vi "maze_v3.vi"   [LabVIEW 2012]
uses:
  <vilib>/NXT/Subs/MotorOutput.ctl
  <vilib>/NXT/Block Support/NXT_InputPort.ctl
  <vilib>/NXT/Dual Mode Library/Motors/MotorReverse.vi
  <vilib>/NXT/Dual Mode Library/Motors/MotorOn.vi
  <vilib>/NXT/Dual Mode Library/Motors/MotorBrake.vi
  <vilib>/NXT/Dual Mode Library/Display/clearDisplay.vi
  <vilib>/NXT/Dual Mode Library/Display/drawText.vi
  <vilib>/NXT/Dual Mode Library/Waits/Wait_Num(msec).vi
  <vilib>/NXT/Dual Mode Library/Display/drawLine.vi
  <vilib>/NXT/Dual Mode Library/Waits/Wait_Num.vi
  <vilib>/NXT/Dual Mode Library/Display/drawNumber.vi
types:
  T1 = typedef "MotorOutput.ctl" = u8
  T2 = typedef "LVHSConnector.ctl" = cluster{"Hardware":string, "Flattened String":string}
  T3 = typedef "NXT_InputPort.ctl" = u8
  T4 = cluster{"x-y*floor(x/y)":i32, "Start X":i16, "x-y*floor(x/y)":i32, i16}
  T5 = cluster{"x":i32, "Start X":i16, "x":i32, "Start X":i16}
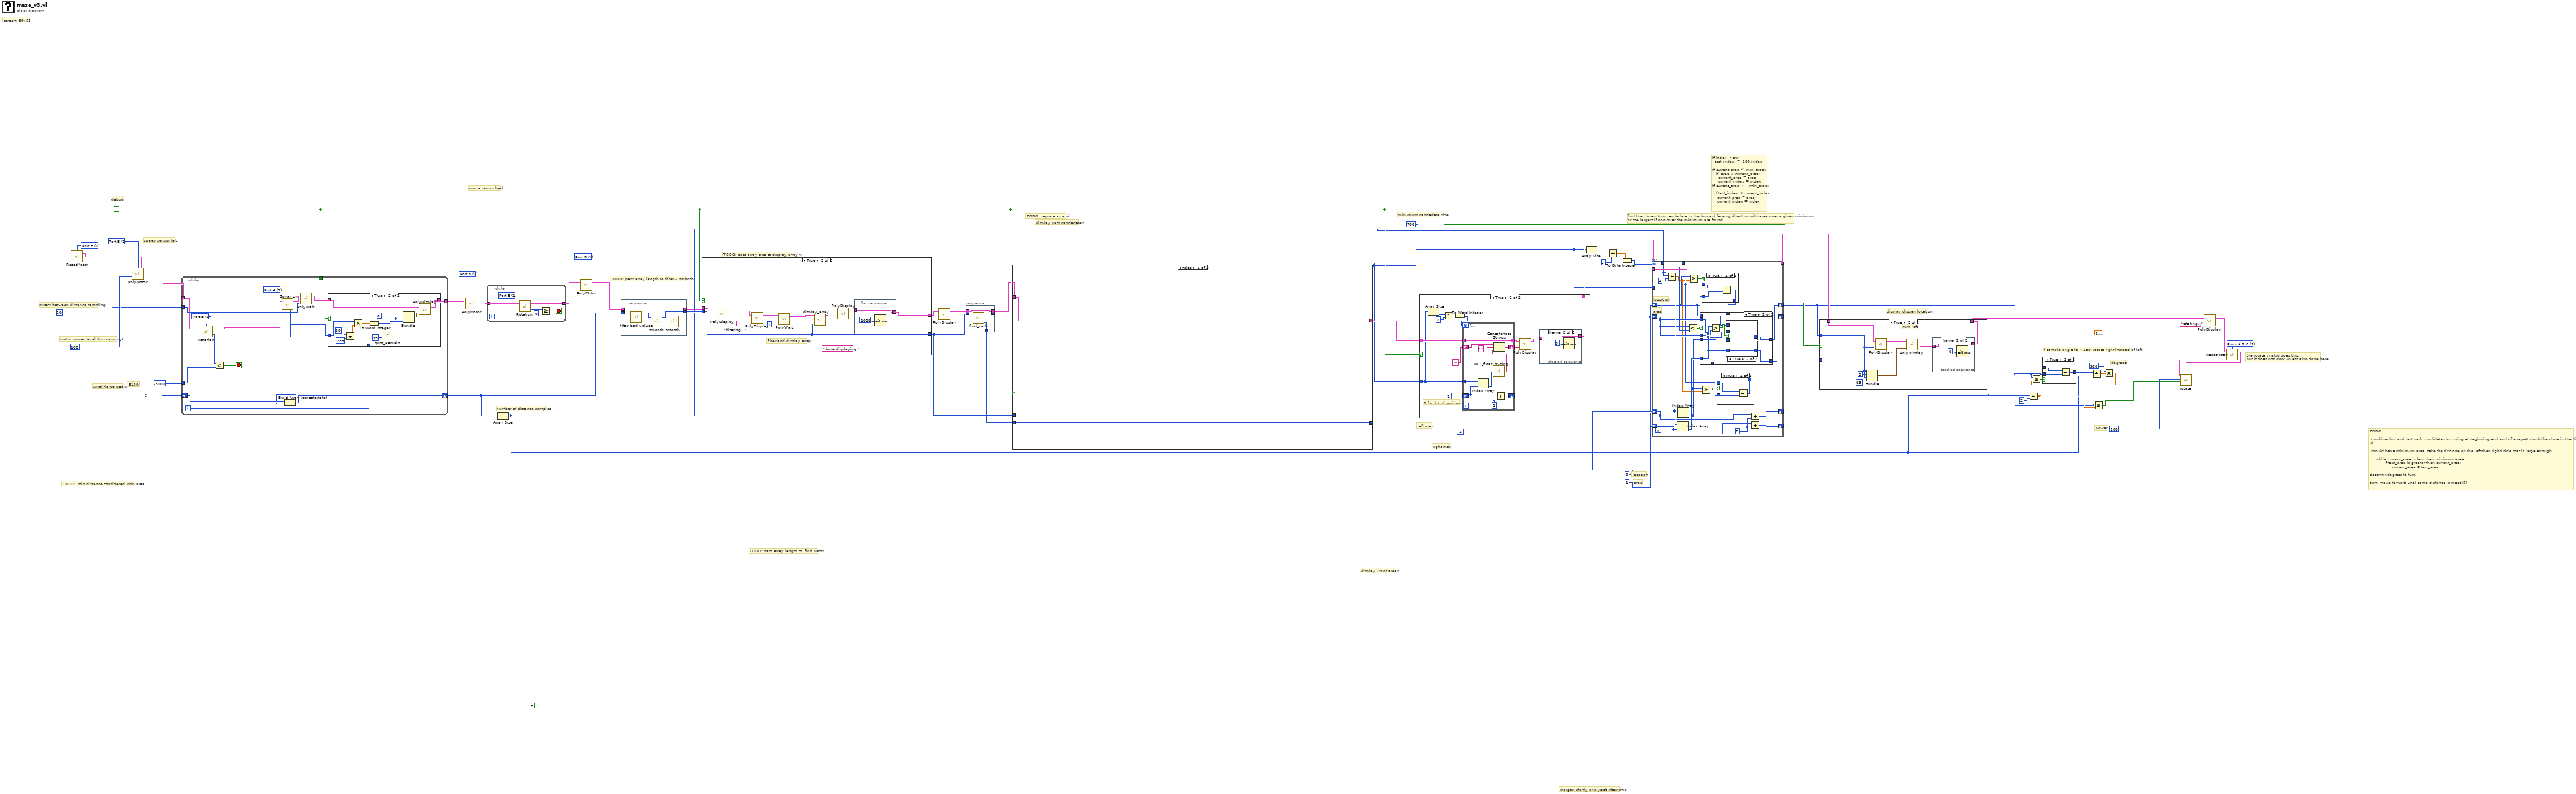
[diagram p0: block diagram]
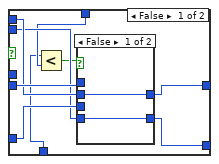
[diagram p9: hidden frame]
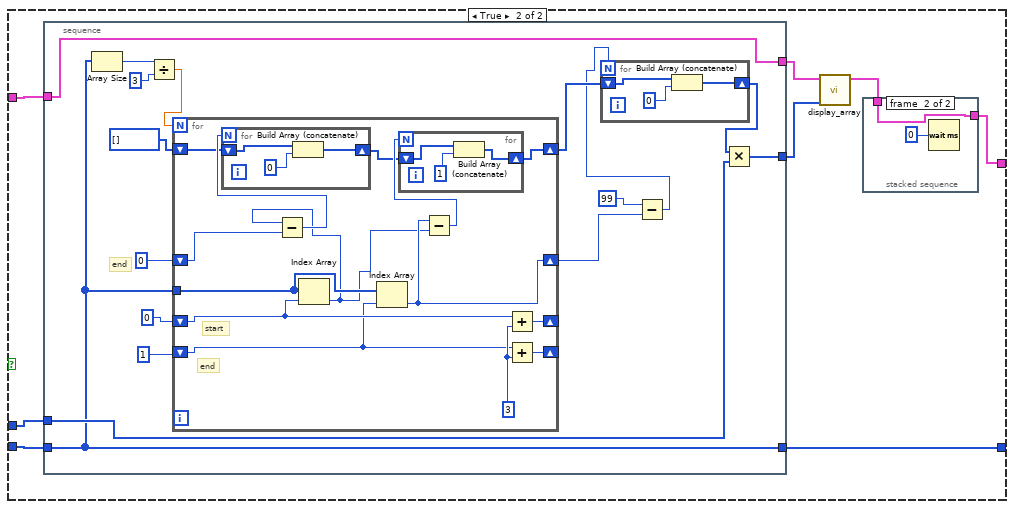
[diagram p13: hidden frame]
diagram:
  w13 = T1 1 items=["Port A"=0, "Port B"=1, "Port C"=2, "Ports A & B"=4, "Ports A & C"=5, "Ports B & C"=6, "as"=3] ("Output Port (All Ports)")
  w14 = T1 1 items=["Port A"=0, "Port B"=1, "Port C"=2, "Ports A & B"=4, "Ports A & C"=5, "Ports B & C"=6, "as"=3] ("Output Port (All Ports)")
  w21 = T1 1 items=["Port A"=0, "Port B"=1, "Port C"=2, "Ports A & B"=4, "Ports A & C"=5, "Ports B & C"=6, "All Ports"=3] ("Port (All Ports)")
  w25 = T1 5 items=["Port A"=0, "Port B"=1, "Port C"=2, "Ports A & B"=4, "Ports A & C"=5, "Ports B & C"=6, "All Ports"=3] ("Port (All Ports)")
  (unwired) 6.283185307179586 ("Pi Multiplied By 2")
  w37 = i16 -1 ("Start X")
  (unwired) FALSE
  w35 = TRUE
  w52 = T1 1 items=["Port A"=0, "Port B"=1, "Port C"=2, "Ports A & B"=4, "Ports A & C"=5, "Ports B & C"=6, "as"=3] ("Output Port (All Ports)")
  # "small-large gears"
  # "-5100"
  # "sweep sensor left"
  # "move sensor back"
  # "if sample angle is > 180, rotate right instead of left"
  # "TODO: pass array length to  find paths"
  # "TODO: pass array size to display array vi"
  # "TODO: pass array length to filter & smooth"
  # "number of distance samples"
  # "the rotate vi also does this,\nbut it does not work unless also done here"
  # "power"
  # "degrees"
  # "display chosen location"
  # "display list of areas"
  # "if index > 50;\n  test_index  =  100-index\n\nif current_area <  min_area:\n   if  area > current_area:\n     current_area = area\n     current_index = index\nif current_area >=  min_area:\n\n  if test_index < current_index:\n    current_area = area\n    current_index = index"
  # "morgan stanly analysist internship"
  # "minumum candedata size"
  # "find the closest turn candedate to the forward faceing direction with area over a given minimum\nor the largest if non over the minimum are found"
  # "TODO:  min distance considered, min area"
  # "msecs between distance sampling"
  # "motor power level (for scanning)"
  # "TODO: seprate as a vi"
  # "TODO:\n\n combine first and last path condidates (occuring at beginning and end of array-->should be done in the 'find paths' vi\n            \n should have minimum area, take the first one on the left(then right) side that is large enough\n\n     while current_area is less then minimum area:\n            if test_area is greator then current_area:\n                  current_area = test_area\n\ndetermindegress to turn\n\nturn, move forward until some distance is meet (?)"
  # "right max"
  # "left max"
  # "display path candedates"
  # "area"
  # "location"
  # "debug"
  # "screen: 99x63"
  n1 = call <vilib>:"ResetMotor.vi"("Port (All Ports)"=w21) -> ("NXT"=w20:T2)  [unwired: 3 in]
  n2 = call-poly <vilib>:"PolyMotor.vi"("Power (75)"=100, "NXT"=w20, "Output Port (All Ports)"=w52) -> ("NXT"=w16:T2)  [unwired: 1 in]
  n3 = while {
    shift-right: [w66] -> w7
    shift-left: i16[] [] -> [w67]
    tunnel: w16 -> [w56]
    tunnel: [w63] -> w12
    tunnel: w35 -> [w62]
    tunnel: 20 -> [w59]
    tunnel: -3100 -> [w55]
    i -> [w60]
    stop <- w57 stop-if-true
    w58 = T1 1 items=["Port A"=0, "Port B"=1, "Port C"=2, "Ports A & B"=4, "Ports A & C"=5, "Ports B & C"=6, "as"=3] ("Output Port (All Ports)")
    w68 = T3 3 items=["Port 1", "Port 2", "Port 3", "Port 4"] ("Port (Port 4)")
    n4 = call <vilib>:"Rotation.vi"("NXT"=w56, "Port (Port A)"=w58) -> ("Angle of Rotation"=w53:i32, "NXT"=w54:T2)  [unwired: 1 in]
    n5 = Less?(x=w53, y=w55) -> (x < y?=w57:bool)
    n6 = call <vilib>:"Sonar_cm.vi"("NXT"=w54, "Port (Port 4)"=w68) -> ("Distance (cm)"=w61:i16, "NXT"=w65:T2)  [unwired: 1 in]
    n7 = Build Array (concatenate)(w67, w61) -> (w66:i16[])
    n8 = call-poly <vilib>:"PolyWait.vi"("Time (100 msec)"=w59, "NXT"=w65) -> ("NXT"=w64:T2)  [unwired: 2 in]
    n9 = case shown="True" w62 {
      tunnel: w64 -> [w69 w79]
      tunnel: [w69 w80] -> w63
      tunnel: w61 -> [_ w78]
      tunnel: w60 -> [_ w71]
      frame False {
      }
      frame True {
        n10 = Divide(x=i16 60 ("Start X"), y=i16 255 ("Start X")) -> (x/y=w76:dbl)
        n11 = Multiply(x=w78, y=w76) -> (x*y=w81:dbl)
        n12 = To Word Integer(number=w81) -> (16bit integer=w73:i16)
        n13 = call <vilib>:"quot_Remain.vi"("y"=i16 99 ("Start X"), "x"=w71) -> ("x-y*floor(x/y)"=w72:i32)  [unwired: 1 out]
        n14 = Bundle("x-y*floor(x/y)"=w72, "Start X"=i16 0, "x-y*floor(x/y)"=w72, w73) -> (w74:T4)  [unwired: 1 in]
        n15 = call-poly <vilib>:"PolyDisplay.vi"("Line Parameters"=w74, "NXT"=w79) -> ("NXT"=w80:T2)  [unwired: 2 in]
      }
    }
  }
  n16 = call-poly <vilib>:"PolyMotor.vi"("NXT"=w12, "Output Port (All Ports)"=w13) -> ("NXT"=w11:T2)  [unwired: 2 in]
  n17 = while {
    tunnel: w11 -> [w88]
    tunnel: [w84] -> w10
    stop <- w83 stop-if-true
    w87 = T1 1 items=["Port A"=0, "Port B"=1, "Port C"=2, "Ports A & B"=4, "Ports A & C"=5, "Ports B & C"=6, "as"=3] ("Output Port (All Ports)")
    n18 = call <vilib>:"Rotation.vi"("NXT"=w88, "Port (Port A)"=w87) -> ("Angle of Rotation"=w86:i32, "NXT"=w84:T2)  [unwired: 1 in]
    n19 = Greater Or Equal?(x=w86, y=0) -> (x >= y?=w83:bool)
  }
  n20 = Array Size(array=w7) -> (size(s)=w17:i32)
  n21 = call-poly <vilib>:"PolyMotor.vi"("NXT"=w10, "Port (All Ports)"=w14) -> ("NXT"=w9:T2)  [unwired: 2 in]
  n22 = stacked-sequence {
    tunnel: w7 -> [w92]
    tunnel: [w90] -> w49
    tunnel: w9 -> [w89]
    tunnel: [w89] -> w8
    frame #0 {
      n23 = call "filter_bad_values.vi"("Array 3"=w92) -> ("Array 4"=w91:i32[])  [unwired: 10 in]
      n24 = call "smooth.vi"("Array"=w91) -> ("Array 2"=w90:i32[])  [unwired: 10 in]
      n25 = call "smooth.vi"() -> ()  [unwired: 11 in, 1 out]
    }
  }
  n26 = case shown="True" w35 {
    tunnel: w8 -> [w94 w100]
    tunnel: w49 -> [w93 w101]
    tunnel: [w94 w98] -> w46
    tunnel: [w93 w101] -> w48
    frame False {
    }
    frame True {
      # "filter and display array"
      n27 = call-poly <vilib>:"PolyDisplay.vi"("NXT"=w100) -> ("NXT"=w99:T2)  [unwired: 3 in]
      n28 = call-poly <vilib>:"PolyDisplay.vi"("Text"="filtering...", "NXT"=w99) -> ("NXT"=w104:T2)  [unwired: 2 in]
      n29 = call-poly <vilib>:"PolyWait.vi"("Time (1 sec)"=i16 1 ("Start X"), "NXT"=w104) -> ("NXT"=w103:T2)  [unwired: 2 in]
      n30 = call "display_array.vi"("array"=w101, "NXT"=w103) -> ("NXT 2"=w96:T2)  [unwired: 9 in]
      n31 = call-poly <vilib>:"PolyDisplay.vi"("Text"="done displaying.", "NXT"=w96) -> ("NXT"=w97:T2)  [unwired: 2 in]
      n32 = flat-sequence {
        tunnel: [w106] -> w98
        tunnel: w97 -> [w106]
        frame #0 {
          n33 = Wait (ms)(milliseconds to wait=u32 1000) -> ()  [unwired: 1 out]
        }
      }
    }
  }
  n34 = call-poly <vilib>:"PolyDisplay.vi"("NXT"=w46) -> ("NXT"=w5:T2)  [unwired: 3 in]
  n35 = stacked-sequence {
    tunnel: w48 -> [w111]
    tunnel: [w110] -> w47
    tunnel: [w109] -> w1
    tunnel: w5 -> [w108]
    tunnel: [w108] -> w4
    frame #0 {
      n36 = call "find_path.vi"("Array"=w111) -> ("debug array"=w110:i32[], "Array 2"=w109:i32[])  [unwired: 9 in]
    }
  }
  n37 = case shown="False" w35 {
    tunnel: w47 -> [w112 w120]
    tunnel: w4 -> [w113 w115]
    tunnel: [w113 w117] -> w42
    tunnel: w48 -> [_ w121]
    tunnel: [w112 w114] -> _
    frame False {
    }
    frame True {
      n38 = stacked-sequence {
        tunnel: w121 -> [w135]
        tunnel: [w134] -> w116
        tunnel: w120 -> [w124]
        tunnel: w115 -> [w125]
        tunnel: [w125] -> w119
        tunnel: [w124] -> w114
        frame #0 {
          # "end"
          n39 = Array Size(array=w124) -> (size(s)=w128:i32)
          n40 = Divide(x=w128, y=3) -> (x/y=w126:dbl)
          n41 = for {
            N: w126 -> [_]
            shift-right: [w155] -> _
            shift-left: i16 0 ("Start X") -> [w152]
            shift-right: [w154] -> _
            shift-left: i16 1 ("Start X") -> [w151]
            shift-right: [w143] -> w133
            shift-left: i16[] [] -> [w145]
            tunnel: w124 -> [w150]
            shift-right: [w148] -> w130
            shift-left: i16 0 ("Start X") -> [w149]
            w156 = 3 ("y")
            # "end"
            # "start"
            n42 = Index Array(array=w150, index=w152) -> (element=w147:i32)
            n43 = Subtract(x=w147, y=w149) -> (x-y=w153:i32)
            n44 = for {
              N: w153 -> [_]
              shift-right: [w161] -> w144
              shift-left: w145 -> [w162]
              n45 = Build Array (concatenate)(w162, i16 0 ("Start X")) -> (w161:i16[])
            }
            n46 = Index Array(array=w150, index=w151) -> (element=w148:i32)
            n47 = Subtract(x=w148, y=w147) -> (x-y=w146:i32)
            n48 = for {
              N: w146 -> [_]
              shift-right: [w157] -> w143
              shift-left: w144 -> [w158]
              n49 = Build Array (concatenate)(w158, i16 1 ("Start X")) -> (w157:i16[])
            }
            n50 = Add(x=w152, y=w156) -> (x+y=w155:i32)
            n51 = Add(x=w151, y=w156) -> (x+y=w154:i32)
          }
          n52 = Subtract(x=i16 99 ("Start X"), y=w130) -> (x-y=w129:i32)
          n53 = for {
            N: w129 -> [_]
            shift-right: [w141] -> w132
            shift-left: w133 -> [w142]
            n54 = Build Array (concatenate)(w142, i16 0 ("Start X")) -> (w141:i16[])
          }
          n55 = Multiply(x=w132, y=w135) -> (x*y=w134:i32[])
        }
      }
      n56 = call "display_array.vi"("array"=w116, "NXT"=w119) -> ("NXT 2"=w118:T2)  [unwired: 9 in]
      n57 = stacked-sequence {
        tunnel: [_ w122] -> w117
        tunnel: w118 -> [_ w122]
        frame #0 {
        }
        frame #1 {
          n58 = Wait (ms)(milliseconds to wait=u32 0) -> ()  [unwired: 1 out]
        }
      }
    }
  }
  n59 = case shown="True" w35 {
    tunnel: w42 -> [w163 w172]
    tunnel: w1 -> [_ w166]
    tunnel: [w163 w165] -> w40
    frame False {
    }
    frame True {
      # "0 for list of positions"
      n60 = Array Size(array=w166) -> (size(s)=w170:i32)
      n61 = Divide(x=w170, y=2) -> (x/y=w168:dbl)
      n62 = To Word Integer(number=w168) -> (16bit integer=w167:i16)
      n63 = for {
        N: w167 -> [_]
        tunnel: w172 -> [w184]
        tunnel: [w184] -> w174
        shift-right: [w185] -> w173
        shift-left: "" ("Text") -> [w187]
        shift-right: [w182] -> _
        shift-left: i16 1 ("Start X") -> [w180]
        tunnel: w166 -> [w179]
        n64 = Index Array(array=w179, index=w180) -> (element=w178:i32)
        n65 = call <vilib>:"NXT_floatToString.vi"("number"=w178) -> ("string"=w186:string)
        n66 = Concatenate Strings(w187, " " ("Text"), w186) -> (w185:string)
        n67 = Add(x=w180, y=i16 2 ("Start X")) -> (x+y=w182:i16)
      }
      n68 = call-poly <vilib>:"PolyDisplay.vi"("Text"=w173, "NXT"=w174) -> ("NXT"=w164:T2)  [unwired: 2 in]
      n69 = stacked-sequence {
        tunnel: w164 -> [_ w176]
        tunnel: [_ w176] -> w165
        frame #0 {
        }
        frame #1 {
          n70 = Wait (ms)(milliseconds to wait=u32 0) -> ()  [unwired: 1 out]
        }
      }
    }
  }
  n71 = Array Size(array=w1) -> (size(s)=w2:i32)
  n72 = Divide(x=w2, y=i16 2 ("Start X")) -> (x/y=w43:dbl)
  n73 = To Byte Integer(number=w43) -> (8bit integer=w41:i8)
  n74 = for {
    N: w41 -> [_]
    tunnel: w1 -> [w209]
    shift-right: [w208] -> _
    shift-left: i16 0 ("Start X") -> [w191]
    shift-right: [w207] -> _
    shift-left: i16 1 ("Start X") -> [w205]
    shift-right: [w200] -> w6
    shift-left: w37 -> [w195]
    shift-right: [w199] -> w36
    shift-left: w37 -> [w192]
    tunnel: w40 -> [w204]
    tunnel: i16 700 ("Start X") -> [w193]
    tunnel: [w204] -> w32
    tunnel: w17 -> [w189]
    w206 = i16 2 ("Start X")
    # "area"
    # "position"
    n75 = Divide(x=w189, y=i16 2 ("Start X")) -> (x/y=w188:dbl)
    n76 = Index Array(array=w209, index=w205) -> (element=w201:i32)
    n77 = Index Array(array=w209, index=w191) -> (element=w194:i32)
    n78 = Less?(x=w192, y=w193) -> (x < y?=w202:bool)
    n79 = Greater Or Equal?(x=w195, y=w188) -> (x >= y?=w203:bool)
    n80 = Greater Or Equal?(x=w194, y=w188) -> (x >= y?=w197:bool)
    n81 = case shown="True" w203 {
      tunnel: w195 -> [w239 w241]
      tunnel: [w239 w242] -> w198
      tunnel: w189 -> [_ w240]
      frame False {
      }
      frame True {
        n82 = Subtract(x=w240, y=w241) -> (x-y=w242:i32)
      }
    }
    n83 = case shown="True" w197 {
      tunnel: w194 -> [w210 w213]
      tunnel: [w210 w212] -> w196
      tunnel: w189 -> [_ w211]
      frame False {
      }
      frame True {
        n84 = Subtract(x=w211, y=w213) -> (x-y=w212:i32)
      }
    }
    n85 = case shown="True" w202 {
      tunnel: w194 -> [w222 w232]
      tunnel: w201 -> [w221 w230]
      tunnel: [w220 w231] -> w200
      tunnel: [w219 w229] -> w199
      tunnel: w198 -> [w216 _]
      tunnel: w196 -> [w215 _]
      tunnel: w195 -> [w218 w228]
      tunnel: w192 -> [w217 w227]
      tunnel: w192 -> [_ w234]
      frame False {
        n86 = Less?(x=w215, y=w216) -> (x < y?=w214:bool)
        n87 = case shown="False" w214 {
          tunnel: w222 -> [_ w226]
          tunnel: w221 -> [_ w225]
          tunnel: [w224 w226] -> w220
          tunnel: [w223 w225] -> w219
          tunnel: w218 -> [w224 _]
          tunnel: w217 -> [w223 _]
          frame False {
          }
          frame True {
          }
        }
      }
      frame True {
        n88 = Greater?(x=w230, y=w234) -> (0:w233:bool)
        n89 = case shown="True" w233 {
          tunnel: w232 -> [_ w238]
          tunnel: [w235 w238] -> w231
          tunnel: w230 -> [_ w237]
          tunnel: [w236 w237] -> w229
          tunnel: w228 -> [w235 _]
          tunnel: w227 -> [w236 _]
          frame False {
          }
          frame True {
          }
        }
      }
    }
    n90 = Add(x=w191, y=w206) -> (x+y=w208:i16)
    n91 = Add(x=w205, y=w206) -> (x+y=w207:i16)
  }
  n92 = case shown="True" w35 {
    tunnel: w6 -> [_ w246]
    tunnel: w32 -> [w243 w248]
    tunnel: [w243 w244] -> w27
    tunnel: w36 -> [_ _]
    frame False {
      # "turn right"
    }
    frame True {
      # "turn left"
      n93 = Bundle("x"=w246, "Start X"=i16 0, "x"=w246, "Start X"=i16 63) -> (w247:T5)  [unwired: 1 in]
      n94 = call-poly <vilib>:"PolyDisplay.vi"("number"=w246, "NXT"=w248) -> ("NXT"=w251:T2)  [unwired: 2 in]
      n95 = call-poly <vilib>:"PolyDisplay.vi"("Line Parameters"=w247, "NXT"=w251) -> ("NXT"=w245:T2)  [unwired: 2 in]
      n96 = stacked-sequence {
        tunnel: w245 -> [_ w252]
        tunnel: [_ w252] -> w244
        frame #0 {
        }
        frame #1 {
          n97 = Wait (ms)(milliseconds to wait=u32 0) -> ()  [unwired: 1 out]
        }
      }
    }
  }
  n98 = Divide(x=w17, y=i16 2 ("Start X")) -> (x/y=w18:dbl)
  n99 = Greater Or Equal?(x=w6, y=w18) -> (x >= y?=w30:bool)
  n100 = case shown="True" w30 {
    tunnel: w6 -> [w254 w256]
    tunnel: [w254 w257] -> w29
    tunnel: w17 -> [_ w255]
    frame False {
    }
    frame True {
      n101 = Subtract(x=w255, y=w256) -> (x-y=w257:i32)
    }
  }
  n102 = Divide(x=w29, y=w17) -> (x/y=w33:dbl)
  n103 = Greater Or Equal?(x=w6, y=w18) -> (x >= y?=w28:bool)
  n104 = Multiply(x=i16 360 ("Start X"), y=w33) -> (x*y=w22:dbl)
  n105 = call-poly <vilib>:"PolyDisplay.vi"("Text"="rotating...", "NXT"=w27) -> ("NXT"=w24:T2)  [unwired: 2 in]
  n106 = call <vilib>:"ResetMotor.vi"("NXT"=w24, "Port (All Ports)"=w25) -> ("NXT"=w23:T2)  [unwired: 2 in]
  n107 = call "rotate.vi"("degrees to  rotate"=w22, "right(T)/left(F)"=w28, "power"=u16 100 ("Max Value"), "NXT 2"=w23) -> ()  [unwired: 7 in, 1 out]
